vi "Write.vi"(6 "Priority":bool, 8 "error in (no error)":errorcluster, 9 "payload":string, 10 "state":string, 11 "queue":refnum<queue>) -> (0 "error out":errorcluster, 3 "queue out":refnum<queue>)   [LabVIEW 2019, in "Simple Queue Message.lvlib"]
uses:
  Simple Queue Message.lvlib
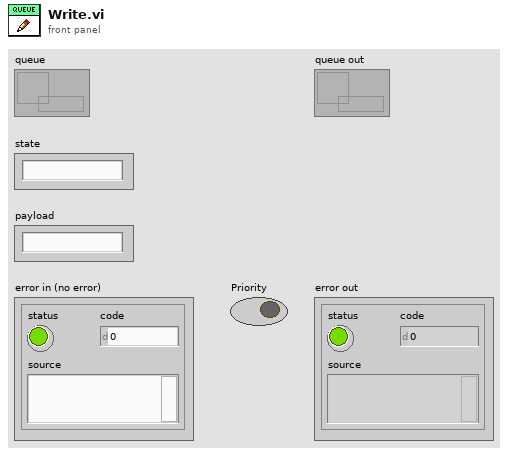
[diagram p1: front panel]
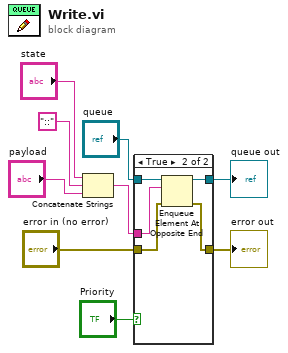
[diagram p0: block diagram]
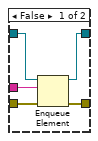
[diagram p2: hidden frame]
diagram:
  n1 = Concatenate Strings("state", "::" ("string"), "payload") -> (w5:string)
  n2 = case shown="True" "Priority" {
    tunnel: "queue" -> [w14 w18]
    tunnel: w5 -> [w13 w19]
    tunnel: "error in (no error)" -> [w12 w17]
    tunnel: [w11 w15] -> w3
    tunnel: [w10 w16] -> w2
    frame False {
      n3 = Enqueue Element(queue=w14, element=w13, error in (no error)=w12) -> (queue out=w11:refnum<queue>, error out=w10:errorcluster)  [unwired: 1 in, 1 out]
    }
    frame True {
      n4 = Enqueue Element At Opposite End(queue=w18, element=w19, error in (no error)=w17) -> (queue out=w15:refnum<queue>, error out=w16:errorcluster)  [unwired: 1 in, 1 out]
    }
  }
  "queue out" <- w3
  "error out" <- w2
